vi "BRig_RT__Case_Idle__State_DispenseWater_pre.vi"(0 "input_dataMTrig":u16[](array[numeric]), 2 "Solenoid_Tcycle_L":u16=300, 3 "Solenoid_Tcycle_R":u16=300, 5 "input_RewCalib__L":bool, 6 "input_RewCalib__R":bool) -> (20 "output_dataMTrig":u16[](array[numeric]), 21 "output_state":T1=enum."DispenseWater")   [LabVIEW 2014]
uses:
  myRIO_Gil_RT__stateList_7,4__NoExp.ctl
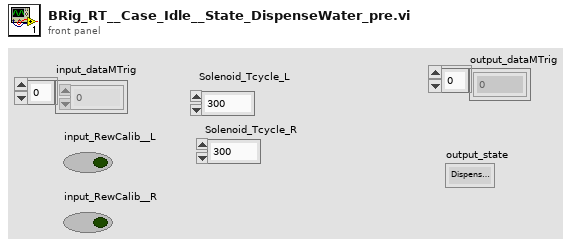
[diagram p1: front panel]
types:
  T1 = typedef "myRIO_Gil_RT__stateList_7,4__NoExp.ctl" = enum16{"Init", "UploadSettings", "Idle", "RewardCalibration_pre", "DispenseWater_pre", "DispenseWater", "DispenseWater_Delay_pre", "DispenseWater_Delay", "TestConnection", "End"}
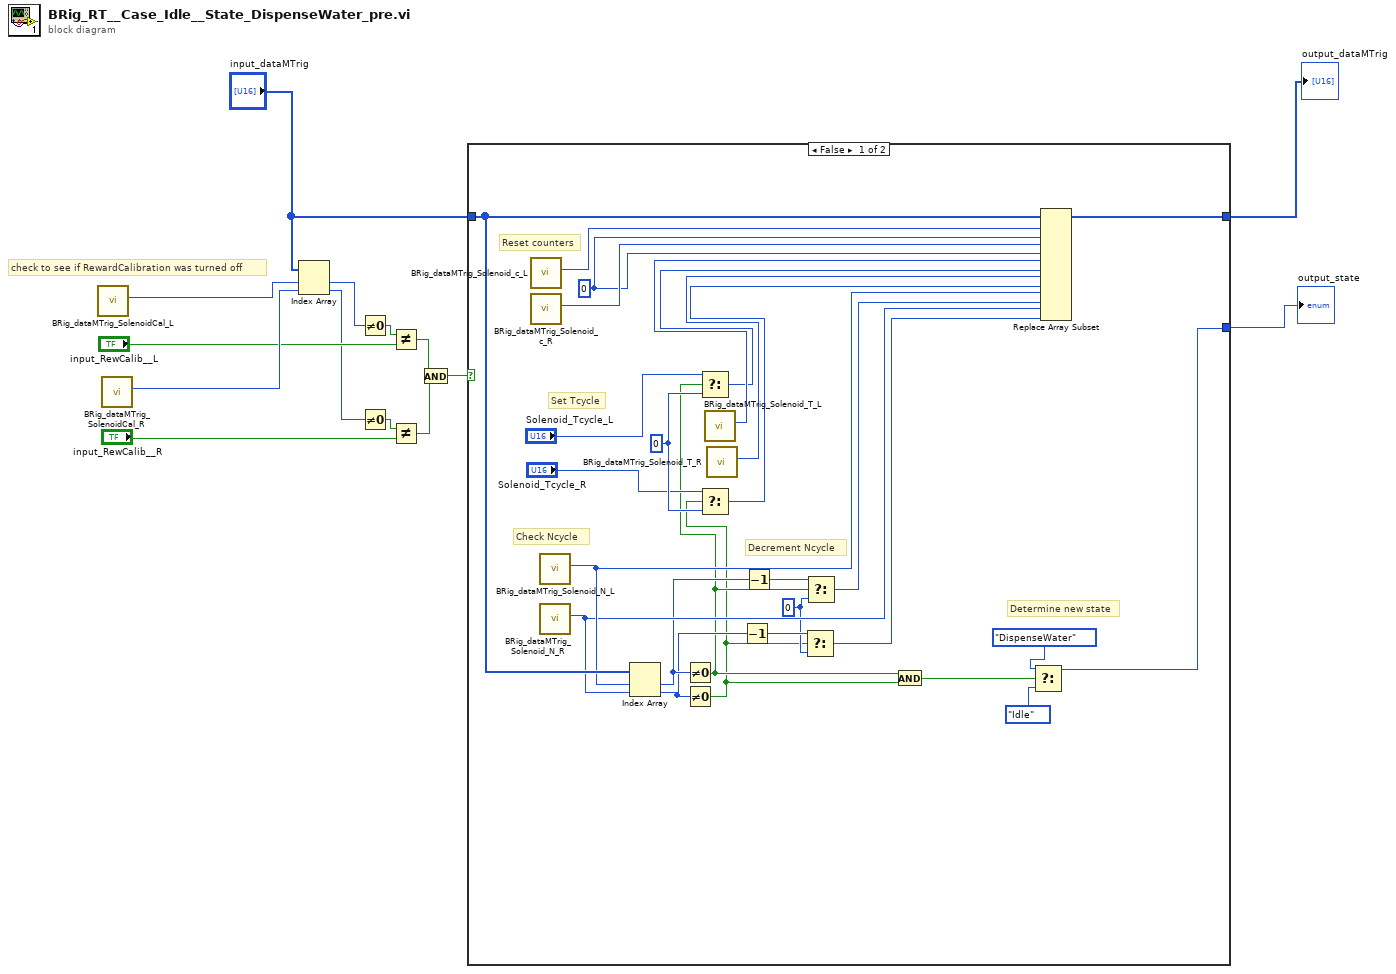
[diagram p0: block diagram]
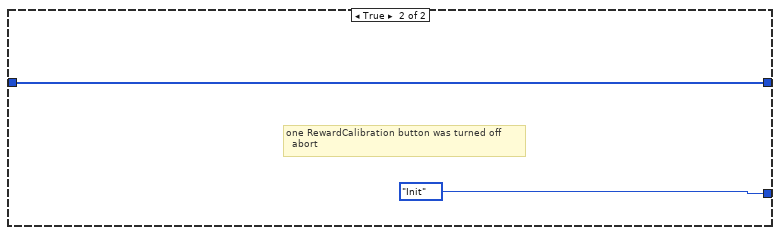
[diagram p2: hidden frame]
diagram:
  # "check to see if RewardCalibration was turned off"
  n1 = call "BRig_dataMTrig_SolenoidCal_L.vi"() -> ("output_SolenoidCal_L"=w12:i32)  [unwired: 11 in]
  n2 = call "BRig_dataMTrig_SolenoidCal_R.vi"() -> ("output_SolenoidCal_R"=w11:i32)  [unwired: 11 in]
  n3 = Index Array(array="input_dataMTrig", index #1=w12, index #2=w11) -> (element #1=w9:u16, element #2=w5:u16)
  n4 = Not Equal To 0?(x=w9) -> (x != 0?=w10:bool)
  n5 = Not Equal To 0?(x=w5) -> (x != 0?=w7:bool)
  n6 = Not Equal?(x=w10, y="input_RewCalib__L") -> (x != y?=w4:bool)
  n7 = Not Equal?(x=w7, y="input_RewCalib__R") -> (x != y?=w3:bool)
  n8 = And(x=w4, y=w3) -> (x .and. y?=w2:bool)
  n9 = case shown="False" w2 {
    tunnel: [w15 w43] -> w14
    tunnel: "input_dataMTrig" -> [w28 w43]
    tunnel: [w18 myRIO_Gil_RT__stateList_7,4__NoExp."Init" ("Enum")] -> w1
    frame False {
      w21 = u16 0 ("f")
      w38 = u16 0 ("f")
      w39 = u16 0 ("new element/subarray")
      # "Determine new state"
      # "Decrement Ncycle"
      # "Check Ncycle"
      # "Set Tcycle"
      # "Reset counters"
      n10 = call "BRig_dataMTrig_Solenoid_c_L.vi"() -> ("output_Solenoid_c_L"=w41:i32)  [unwired: 11 in]
      n11 = call "BRig_dataMTrig_Solenoid_c_R.vi"() -> ("output_Solenoid_c_R"=w40:i32)  [unwired: 11 in]
      n12 = call "BRig_dataMTrig_Solenoid_N_L.vi"() -> ("output_Solenoid_N_L"=w27:i32)  [unwired: 11 in]
      n13 = call "BRig_dataMTrig_Solenoid_N_R.vi"() -> ("output_Solenoid_N_R"=w26:i32)  [unwired: 11 in]
      n14 = Index Array(array=w28, index #1=w27, index #2=w26) -> (element #1=w25:u16, element #2=w23:u16)
      n15 = Not Equal To 0?(x=w25) -> (x != 0?=w17:bool)
      n16 = Not Equal To 0?(x=w23) -> (x != 0?=w16:bool)
      n17 = Select(t="Solenoid_Tcycle_L", s=w17, f=w38) -> (s? t:f=w34:u16)
      n18 = Select(t="Solenoid_Tcycle_R", s=w16, f=w38) -> (s? t:f=w32:u16)
      n19 = call "BRig_dataMTrig_Solenoid_T_L.vi"() -> ("output_Solenoid_T_L"=w35:i32)  [unwired: 11 in]
      n20 = call "BRig_dataMTrig_Solenoid_T_R.vi"() -> ("output_Solenoid_T_R"=w33:i32)  [unwired: 11 in]
      n21 = Decrement(x=w23) -> (x-1=w22:u16)
      n22 = Decrement(x=w25) -> (x-1=w24:u16)
      n23 = Select(t=w22, s=w16, f=w21) -> (s? t:f=w19:u16)
      n24 = Select(t=w24, s=w17, f=w21) -> (s? t:f=w20:u16)
      n25 = And(x=w17, y=w16) -> (x .and. y?=w31:bool)
      n26 = Select(t=myRIO_Gil_RT__stateList_7,4__NoExp."DispenseWater" ("Enum"), s=w31, f=myRIO_Gil_RT__stateList_7,4__NoExp."Idle" ("Enum")) -> (s? t:f=w18:T1)
      n27 = Replace Array Subset(array=w28, new element #1=w39, index #1=w41, new element #2=w39, index #2=w40, new element #3=w34, index #3=w35, new element #4=w32, index #4=w33, new element #5=w20, index #5=w27, new element #6=w19, index #6=w26) -> (w15:u16[])
    }
    frame True {
      # "one RewardCalibration button was turned off\n  abort"
    }
  }
  "output_dataMTrig" <- w14
  "output_state" <- w1
